vi "Rename Constructor.vi"(6 "All Descendents":refnum<vi>[](array[refnum]), 11 "QControl Creation in":refnum<class "QControl Creation.lvclass">) -> (0 "error out":errorcluster, 2 "Constructor Method VI out":refnum<vi>, 3 "QControl Creation out":refnum<class "QControl Creation.lvclass">)   [LabVIEW 2015, in "QControl Creation.lvclass"]
doc: "<b> </b> <b> </b>\n©2016 Q Software Innovations, LLC (QSI)\nwritten by Quentin Alldredge\nproduced in LabVIEW 2015\n\nsupport@qsoftwareinnovations.com\nwww.qsoftwareinnovations.com\n\nAll rights reserved.\n\nRedistribution and use in source and binary forms, with or without modification, are permitted provided that the following conditions are met:\n\n * Redistributions of source code must retain the above copyright notice, this list of conditions and the following disclaimer.\n * Redistributions in binary form must reproduce the above copyright notice, this list of conditions and the following disclaimer in the documentation and/or other materials provided with the distribution.\n * Neither the name of Q Software Innovations, LLC. nor the names of its contributors may be used to endorse or promote products derived from this software without specific prior written permission.\n\nTHIS SOFTWARE IS PROVIDED BY THE COPYRIGHT HOLDERS AND CONTRIBUTORS \"AS IS\" AND ANY EXPRESS OR IMPLIED WARRANTIES, INCLUDING, BUT NOT LIMITED TO, THE IMPLIED WARRANTIES OF MERCHANTABILITY AND FITNESS FOR A PARTICULAR PURPOSE ARE DISCLAIMED. IN NO EVENT SHALL THE COPYRIGHT OWNER OR CONTRIBUTORS BE LIABLE FOR ANY DIRECT, INDIRECT, INCIDENTAL, SPECIAL, EXEMPLARY, OR CONSEQUENTIAL DAMAGES (INCLUDING, BUT NOT LIMITED TO, PROCUREMENT OF SUBSTITUTE GOODS OR SERVICES; LOSS OF USE, DATA, OR PROFITS; OR BUSINESS INTERRUPTION) HOWEVER CAUSED AND ON ANY THEORY OF LIABILITY, WHETHER IN CONTRACT, STRICT LIABILITY, OR TORT (INCLUDING NEGLIGENCE OR OTHERWISE) ARISING IN ANY WAY OUT OF THE USE OF THIS SOFTWARE, EVEN IF ADVISED OF THE POSSIBILITY OF SUCH DAMAGE."
uses:
  QControl Creation.lvclass
  QControl Creation.lvclass/QControl Creation.ctl
  New QControl Info/New QControl Info.lvclass/New QControl Info.ctl
  New QControl Info/Read QControl Class Name.vi
  <vilib>/Utility/error.llb/Error Cluster From Error Code.vi
  <vilib>/ErrorRing/Error Ring.xnode
  New QControl Info/New QControl Info.lvclass
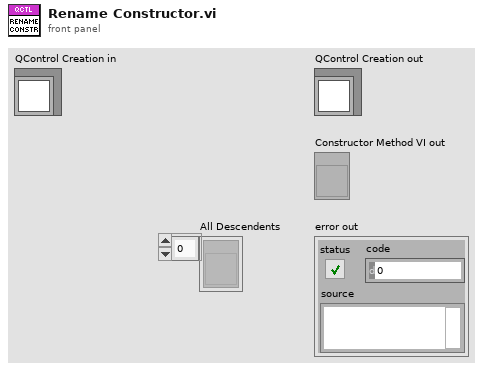
[diagram p1: front panel]
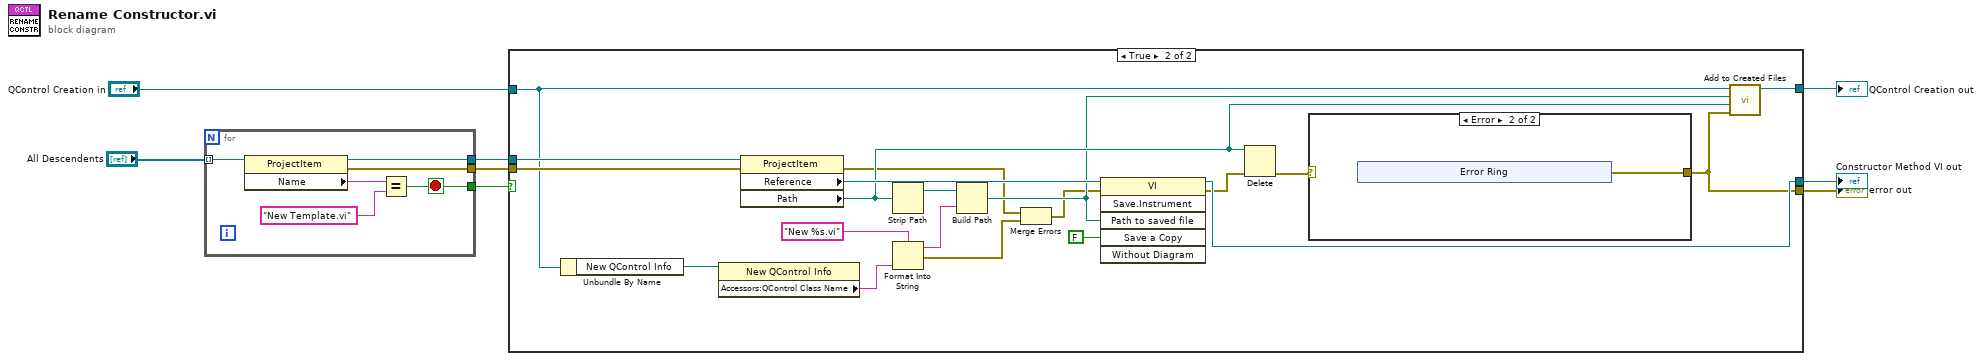
[diagram p0: block diagram]
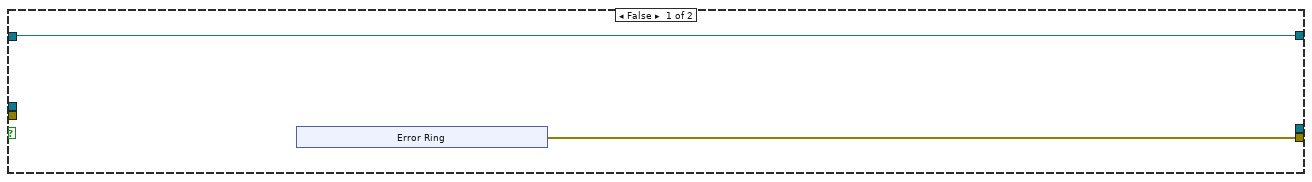
[diagram p2: hidden frame]
diagram:
  n1 = for {
    tunnel: "All Descendents" -> [w14] mode=indexing
    tunnel: [w11] -> w5
    tunnel: [w10] -> w4
    tunnel: [w9] -> w3
    stop <- w10 stop-if-true
    n2 = property class="ProjectItem"(reference=w14) -> (reference out=w11:refnum<vi>, error out=w9:errorcluster, "Name"=w13:string)  [unwired: 1 in]
    n3 = Equal?(x=w13, y="New Template.vi" ("format string")) -> (x = y?=w10:bool)
  }
  n4 = case shown="True" w4 {
    tunnel: [_ w41] -> w8
    tunnel: [w16 w28] -> w7
    tunnel: w5 -> [_ w34]
    tunnel: w3 -> [_ w33]
    tunnel: "QControl Creation in" -> [w15 w31]
    tunnel: [w15 w27] -> w1
    frame False {
      n5 = xnode "Error Ring"() -> ("error out"=w16:errorcluster)
    }
    frame True {
      n6 = Unbundle By Name(w31) -> ("New QControl Info"=w32:refnum<data-value>)
      n7 = property class="New QControl Info"(reference=w32) -> ("Accessors:QControl Class Name"=w23:string)  [unwired: 1 in, 2 out]
      n8 = property class="ProjectItem"(reference=w34, error in=w33) -> (error out=w26:errorcluster, "Reference"=w35:refnum<vi>, "Path"=w30:path)  [unwired: 1 out]
      n9 = Strip Path(path=w30) -> (stripped path=w40:path)  [unwired: 1 out]
      n10 = Format Into String(format string="New %s.vi", w23) -> (resulting string=w38:string, error out=w24:errorcluster)  [unwired: 2 in]
      n11 = Build Path(base path=w40, name or relative path=w38) -> (appended path=w29:path)
      n12 = Merge Errors(w26, w24) -> (w25:errorcluster)
      n13 = invoke class="VI" method="Save.Instrument"(reference=w35, error in=w25, "Path to saved file"=w29, "Save a Copy"=FALSE) -> (reference out=w41:refnum<vi>, error out=w36:errorcluster)  [unwired: 2 in, 4 out]
      n14 = Delete(path (use dialog)=w30, error in=w36) -> (error out=w22:errorcluster)  [unwired: 3 in, 2 out]
      n15 = case shown="Error" w22 {
        selector: w22 -> [w42 _]
        tunnel: [w42 w43] -> w28
        frame No Error {
        }
        frame Error {
          n16 = xnode "Error Ring"() -> ("error out"=w43:errorcluster)
        }
      }
      n17 = call "Add to Created Files.vi"("error in (no error)"=w28, "Path to Replace (\"\")"=w30, "Path to Add"=w29, "QControl Creation in"=w31) -> ("QControl Creation out"=w27:refnum<class "QControl Creation.lvclass">)  [unwired: 7 in]
    }
  }
  "Constructor Method VI out" <- w8
  "error out" <- w7
  "QControl Creation out" <- w1
